vi "2025_day11 recursive search.vi"(6 "End Device Label":string, 8 "# of valid paths in":i32, 9 "Dev idx":i32, 10 "path history in":string[](array[string]), 11 "Data in":string[][](array[string])) -> (0 "# of valid paths out":i32, 2 "path history out":string[](array[string]), 3 "Data out":string[][](array[string]))   [LabVIEW 2025]
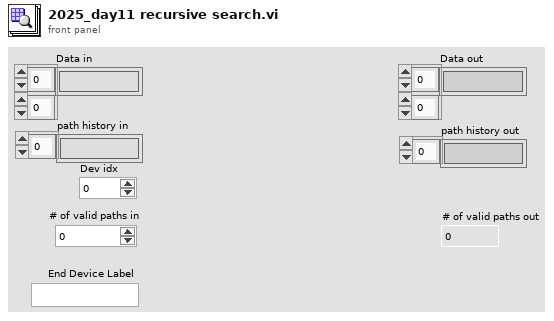
[diagram p1: front panel]
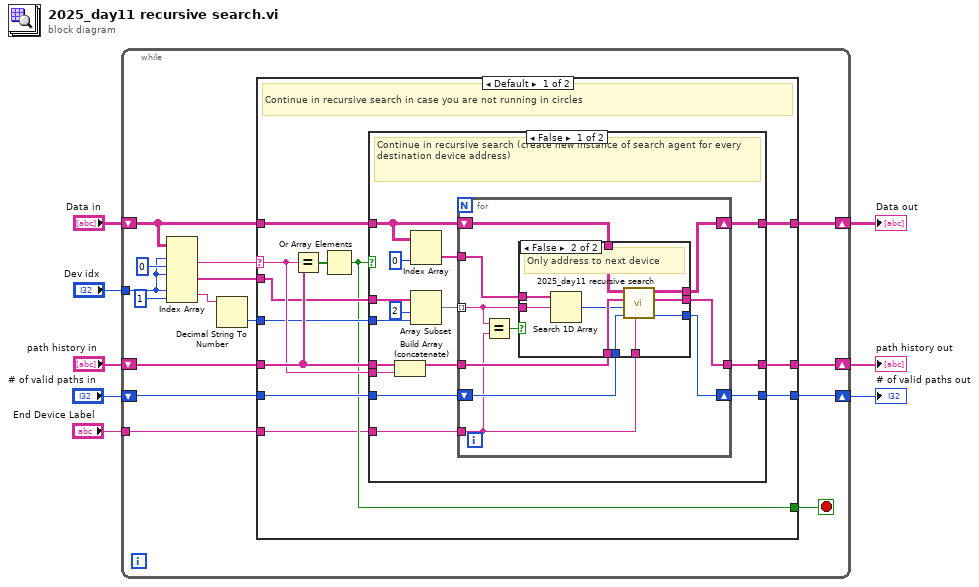
[diagram p0: block diagram]
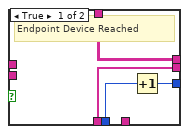
[diagram p2: hidden frame]
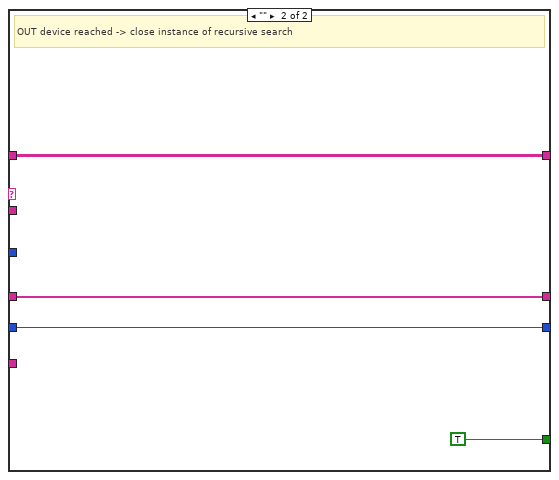
[diagram p4: hidden frame]
diagram:
  n1 = while {
    shift-right: [w19] -> w6
    shift-left: "Data in" -> [w18]
    shift-right: [w21] -> w8
    shift-left: "# of valid paths in" -> [w20]
    tunnel: "Dev idx" -> [w10]
    shift-right: [w22] -> w7
    shift-left: "path history in" -> [w23]
    tunnel: "End Device Label" -> [w9]
    stop <- w17 stop-if-true
    n2 = Index Array(array=w18, index (row) #1=w10, index (col) #1=0 ("disabled index (col)"), index (row) #2=w10, index (row) #3=w10, index (col) #3=1 ("disabled index (col)")) -> (element #1=w15:string, element #2=w12:string[], element #3=w11:string)  [unwired: 1 in]
    n3 = Decimal String To Number(string=w11) -> (number=w14:i32)  [unwired: 2 in, 1 out]
    n4 = case shown="Default" w15 {
      selector: w15 -> [w34 _]
      tunnel: w23 -> [w35 w78]
      tunnel: [w25 w78] -> w22
      tunnel: [w32 w81] -> w21
      tunnel: w20 -> [w31 w81]
      tunnel: [w27 w80] -> w19
      tunnel: w18 -> [w26 w80]
      tunnel: [w28 TRUE] -> w17
      tunnel: w12 -> [w30 _]
      tunnel: w14 -> [w29 _]
      tunnel: w9 -> [w24 _]
      frame Default {
        # "Continue in recursive search in case you are not running in circles"
        n5 = Equal?(x=w34, y=w35) -> (x = y?=w33:bool[])
        n6 = Or Array Elements(Boolean array=w33) -> (logical OR=w28:bool)
        n7 = case shown="False" w28 {
          tunnel: w35 -> [w50 w76]
          tunnel: w34 -> [w49 _]
          tunnel: [w47 w75] -> w32
          tunnel: w31 -> [w48 w75]
          tunnel: w30 -> [w45 _]
          tunnel: w29 -> [w44 _]
          tunnel: [w41 w77] -> w27
          tunnel: w26 -> [w39 w77]
          tunnel: [w40 w76] -> w25
          tunnel: w24 -> [w36 _]
          frame False {
            # "Continue in recursive search (create new instance of search agent for every destination device address)"
            n8 = Build Array (concatenate)(w50, w49) -> (w42:string[])
            n9 = Index Array(array=w39, index (col)=0 ("disabled index (col)")) -> (element=w37:string[])  [unwired: 1 in]
            n10 = Array Subset(array=w45, index=2, length=w44) -> (w43:string[])
            n11 = for {
              shift-right: [w55] -> w47
              shift-left: w48 -> [w56]
              tunnel: w43 -> [w53] mode=indexing
              shift-right: [w59] -> w41
              shift-left: w39 -> [w60]
              tunnel: w37 -> [w54]
              tunnel: w42 -> [w58]
              tunnel: [w57] -> w40
              tunnel: w36 -> [w51]
              n12 = Equal?(x=w53, y=w51) -> (x = y?=w52:bool)
              n13 = case shown="False" w52 {
                tunnel: w60 -> [w64 w74]
                tunnel: [w64 w73] -> w59
                tunnel: w58 -> [w63 w72]
                tunnel: [w63 w71] -> w57
                tunnel: w54 -> [_ w69]
                tunnel: w56 -> [w61 w67]
                tunnel: [w62 w66] -> w55
                tunnel: w53 -> [_ w70]
                tunnel: w51 -> [_ w65]
                frame True {
                  # "Endpoint Device Reached"
                  n14 = Increment(x=w61) -> (x+1=w62:i32)
                }
                frame False {
                  # "Only address to next device"
                  n15 = Search 1D Array(1D array=w69, element=w70) -> (index of element=w68:i32)  [unwired: 1 in]
                  n16 = call "2025_day11 recursive search.vi"("End Device Label"=w65, "# of valid paths in"=w67, "Dev idx"=w68, "path history in"=w72, "Data in"=w74) -> ("# of valid paths out"=w66:i32, "path history out"=w71:string[], "Data out"=w73:string[][])  [unwired: 4 in]
                }
              }
            }
          }
          frame True {
            # "Running in circles -> STOP this branch of\nrecursive search"
          }
        }
      }
      frame "" {
        # "OUT device reached -> close instance of recursive search"
      }
    }
  }
  "# of valid paths out" <- w8
  "path history out" <- w7
  "Data out" <- w6
